vi "bh3_open_bt_cnx.vi"(8 "error in (no error)":errorcluster, 10 "bt time limit ms (5000)":i32=5000, 11 "device name":string="BH BHT011176") -> (0 "error out":errorcluster, 3 "bt connection ID":refnum<k31>)   [LabVIEW 2013]
panel:
  out "bt devicce info":cluster{"Address":string, "Device Name":string}
  out "bt device list":T1(array[cluster])
  out "bt device service list":T2(array[cluster])
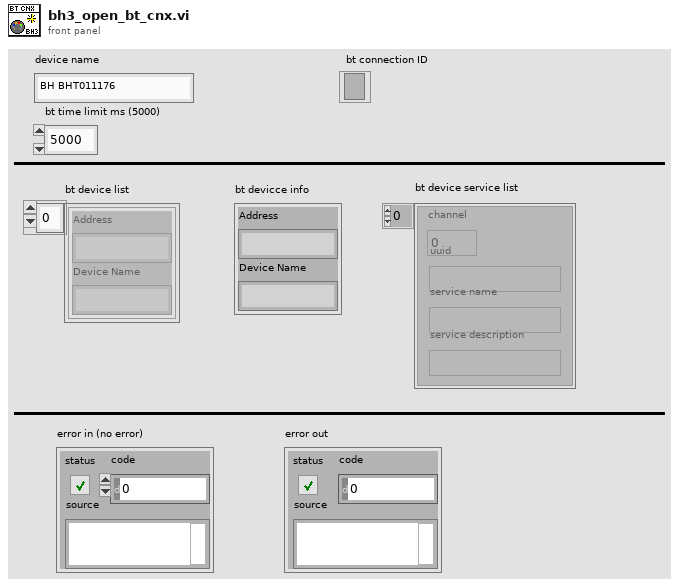
[diagram p1: front panel]
types:
  T1 = cluster{"Address":string, "Device Name":string}[]
  T2 = cluster{"channel":u16, "uuid":string, "service name":string, "service description":string}[]
  T3 = cluster{"channel":u16, "uuid":string, "service name":string, "service description":string}
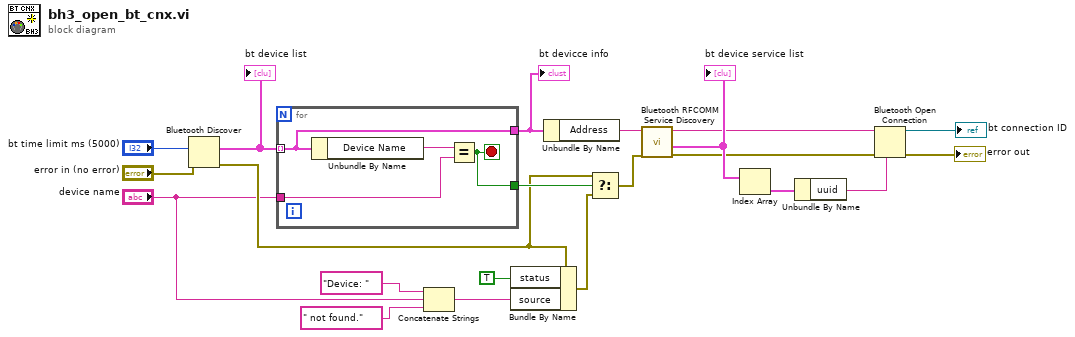
[diagram p0: block diagram]
diagram:
  n1 = Bluetooth Discover(8:"error in (no error)", 10:"bt time limit ms (5000)") -> (0:w7:errorcluster, 2:w21:T1)  [unwired: 1 out]
  "bt device list" <- w21
  n2 = for {
    tunnel: w21 -> [w24] mode=indexing
    tunnel: [w24] -> w12
    tunnel: "device name" -> [w23]
    tunnel: [w22] -> w8
    stop <- w22 stop-if-true
    n3 = Unbundle By Name(w24) -> ("Device Name"=w25:string)
    n4 = Equal?(x=w25, y=w23) -> (x = y?=w22:bool)
  }
  "bt devicce info" <- w12
  n5 = Concatenate Strings("Device: " ("string"), "device name", " not found." ("string")) -> (w1:string)
  n6 = Bundle By Name(cluster=w7, "status"=TRUE, "source"=w1) -> (w6:errorcluster)
  n7 = Unbundle By Name(w12) -> ("Address"=w20:string)
  n8 = Select(t=w7, s=w8, f=w6) -> (s? t:f=w9:errorcluster)
  n9 = call <vilib>:"Bluetooth RFCOMM Service Discovery.vi"("error in (no error)"=w9, "address in"=w20) -> ("error out"=w15:errorcluster, "service list"=w19:T2, "address out"=w18:string)  [unwired: 2 in, 1 out]
  "bt device service list" <- w19
  n10 = Index Array(array=w19) -> (element=w17:T3)  [unwired: 1 in]
  n11 = Unbundle By Name(w17) -> ("uuid"=w16:string)
  n12 = Bluetooth Open Connection(6:w16, 8:w15, 11:w18) -> (0:→"error out":errorcluster, 3:→"bt connection ID":refnum<k31>)  [unwired: 2 in]
